vi "Set Permanent SysEnvVariable.vi"(8 "error in (no error)":errorcluster, 10 "Value":string, 11 "Key":string) -> (0 "error out":errorcluster, 3 "standard output":string)   [LabVIEW 2017]
doc: "Sets a Windows environment variable permanently by running setx, so the value survives a restart. The value may be given literally or as a reference to another environment variable."
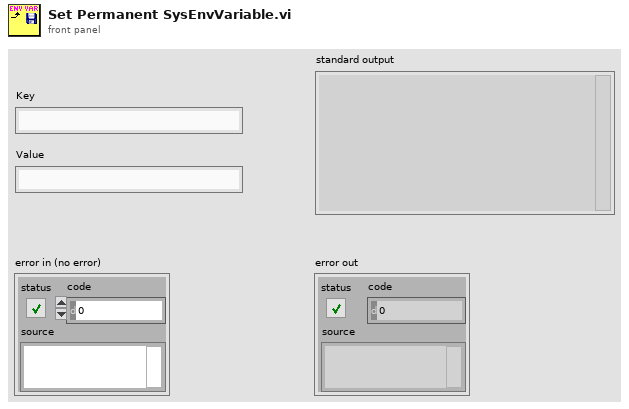
[diagram p1: front panel]
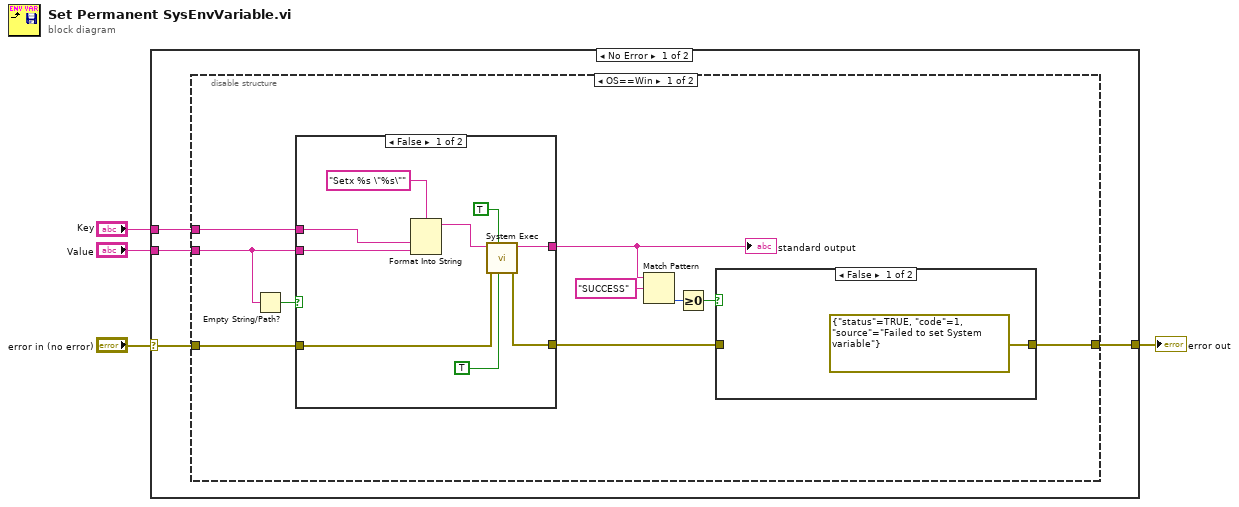
[diagram p0: block diagram]
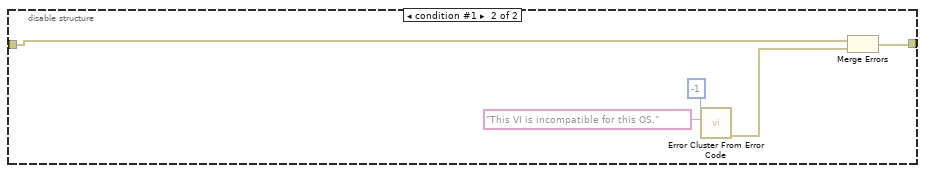
[diagram p4: hidden frame]
diagram:
  n1 = case shown="No Error" "error in (no error)" {
    selector: "error in (no error)" -> [w8 w36]
    tunnel: "Value" -> [w7 _]
    tunnel: [w6 w36] -> w2
    tunnel: "Key" -> [w5 _]
    frame No Error {
      n2 = disable-structure shown="OS==Win" {
        disable-tunnel: w8 -> [w18 w31]
        disable-tunnel: w7 -> [w15 _]
        disable-tunnel: [w10 w32] -> w6
        disable-tunnel: w5 -> [w9 _]
        frame condition #0 (active) {
          n3 = Empty String/Path?(string/path=w15) -> (empty?=w14:bool)
          n4 = case shown="False" w14 {
            tunnel: w18 -> [w29 w30]
            tunnel: [w28 w30] -> w13
            tunnel: [w27 _] -> w17
            tunnel: w15 -> [w25 _]
            tunnel: w9 -> [w24 _]
            frame False {
              n5 = Format Into String(format string="Setx %s \"%s\"" ("string"), w24, w25) -> (resulting string=w23:string)  [unwired: 2 in, 1 out]
              n6 = call <vilib>:"System Exec.vi"("run minimized? (F)"=TRUE, "wait until completion? (T)"=TRUE, "error in (no error)"=w29, "command line"=w23) -> ("error out"=w28:errorcluster, "standard output"=w27:string)  [unwired: 4 in, 2 out]
            }
            frame True {
            }
          }
          "standard output" <- w17
          n7 = Match Pattern(string=w17, regular expression="SUCCESS") -> (offset past match=w12:i32)  [unwired: 1 in, 3 out]
          n8 = Greater Or Equal To 0?(x=w12) -> (x >= 0?=w11:bool)
          n9 = case shown="False" w11 {
            tunnel: w13 -> [_ w20]
            tunnel: [errorcluster {"status"=TRUE, "code"=1, "source"="Failed to set System variable"} ("error IO") w20] -> w10
            frame False {
            }
            frame True {
            }
          }
        }
        frame condition #1 {
          n10 = call <vilib>:"Error Cluster From Error Code.vi"("error message (\"\")"="This VI is incompatible for this OS." ("error message (\"\")"), "error code (0)"=-1) -> ("error out"=w35:errorcluster)  [unwired: 7 in]
          n11 = Merge Errors(w31, w35) -> (w32:errorcluster)
        }
      }
    }
    frame Error {
    }
  }
  "error out" <- w2
